vi "read_v2.vi"(8 "error in (no error)":errorcluster, 9 "Boolean 2":bool, 10 "Boolean":bool, 11 "VISA resource name":refnum<visa-resource-name>) -> (0 "error out":errorcluster, 1 "XY Graph":cluster{"Y":dbl[], "Y":dbl[]}(graph), 2 "Waveform Graph":waveform(dbl)[](graph), 3 "VISA resource name out":refnum<visa-resource-name>)   [LabVIEW 2021]
uses:
  <instrlib>/Tektronix TDS 200 1000 2000 Series/Tektronix TDS 200 1000 2000 Series.lvlib
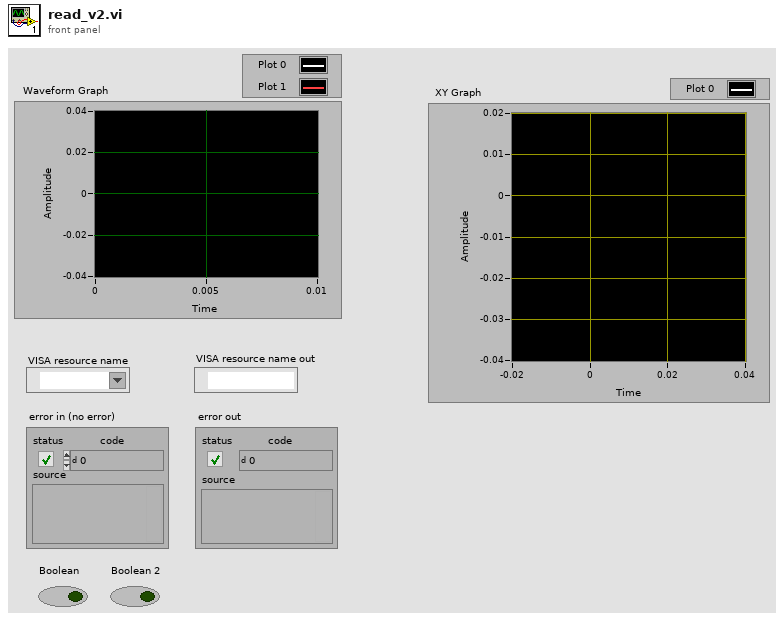
[diagram p1: front panel]
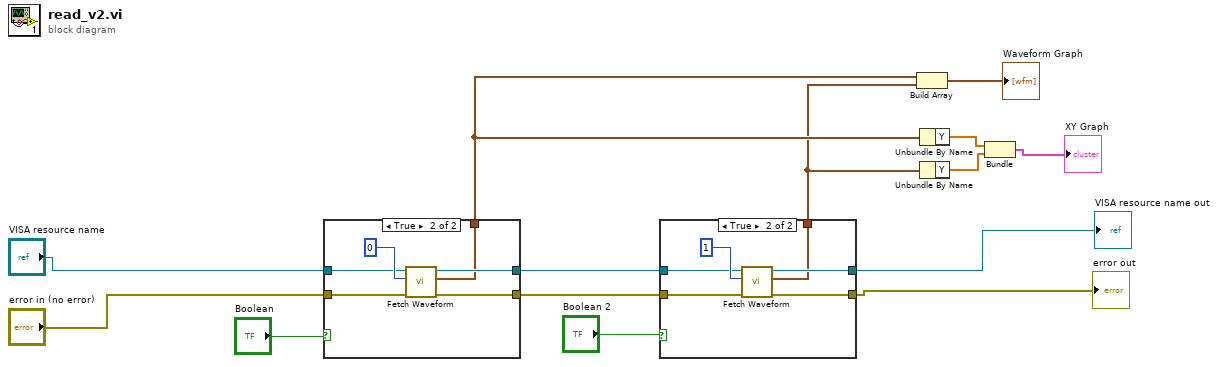
[diagram p0: block diagram]
diagram:
  n1 = case shown="True" "Boolean" {
    tunnel: "VISA resource name" -> [w16 w21]
    tunnel: "error in (no error)" -> [w15 w20]
    tunnel: [w16 w19] -> w12
    tunnel: [w15 w18] -> w11
    tunnel: [_ w17] -> w5
    frame False {
    }
    frame True {
      n2 = call <instrlib>:"Fetch Waveform.vi"("error in (no error)"=w20, "Source (0: Channel 1)"=0, "VISA resource name"=w21) -> ("error out"=w18:errorcluster, "Waveform Data"=w17:waveform(dbl), "VISA resource name out"=w19:refnum<visa-resource-name>)  [unwired: 6 in]
    }
  }
  n3 = case shown="True" "Boolean 2" {
    tunnel: w12 -> [w24 w29]
    tunnel: w11 -> [w23 w28]
    tunnel: [w24 w27] -> w10
    tunnel: [w23 w26] -> w9
    tunnel: [_ w25] -> w4
    frame False {
    }
    frame True {
      n4 = call <instrlib>:"Fetch Waveform.vi"("error in (no error)"=w28, "Source (0: Channel 1)"=1, "VISA resource name"=w29) -> ("error out"=w26:errorcluster, "Waveform Data"=w25:waveform(dbl), "VISA resource name out"=w27:refnum<visa-resource-name>)  [unwired: 6 in]
    }
  }
  "error out" <- w9
  "VISA resource name out" <- w10
  n5 = Build Array(w5, w4) -> (→"Waveform Graph":waveform(dbl)[])
  n6 = Unbundle By Name(w5) -> ("Y"=w3:dbl[])
  n7 = Unbundle By Name(w4) -> ("Y"=w2:dbl[])
  n8 = Bundle("Y"=w3, "Y"=w2) -> (→"XY Graph":cluster{"Y":dbl[], "Y":dbl[]})  [unwired: 1 in]
